vi "MV3D RGBD Release.vi"() -> (3 "function return":i32)   [LabVIEW 2015, in "Mv3dRgbd.lvlib"]
doc: "MV3D_RGBD_API MV3D_RGBD_STATUS MV3D_RGBD_Release();"
uses:
  <userlib>/Mv3dRgbd/Mv3dRgbd.lvlib
  <userlib>/Mv3dRgbd/Mv3dRgbd.dll
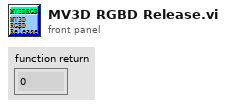
[diagram p1: front panel]
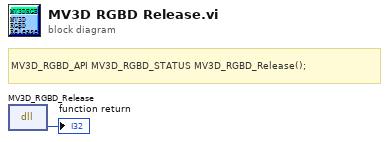
[diagram p0: block diagram]
diagram:
  # "MV3D_RGBD_API MV3D_RGBD_STATUS MV3D_RGBD_Release();"
  n1 = dll-call lib="C:/Program Files (x86)/National Instruments/LabVIEW 2015/user.lib/Mv3dRgbd/Mv3dRgbd.*" fn="MV3D_RGBD_Release"() -> (→"function return":i32)  [unwired: 3 in, 2 out]
